vi "Update Plugin Status.vi"(8 "error in (no error)":errorcluster, 11 "CIF_UI in":refnum<class "CIF_UI.lvclass">) -> (0 "error out":errorcluster, 3 "CIF_UI out":refnum<class "CIF_UI.lvclass">)   [LabVIEW 2021, in "CIF_UI.lvclass"]
uses:
  CIF_UI.lvclass
  CIF_UI.lvclass/CIF_UI.ctl
  <vilib>/Utility/miscctls.llb/LVMapReplaceAction.ctl
  <vilib>/Utility/error.llb/Clear Errors.vi
  <vilib>/gRPC/LabVIEW gRPC Library/Client API/Close Client.vi
  CIFPluginManager/gRPC/CIF_Manager_Client_Wrapper/CIFManagerClientWrapper.lvlib
  CIFCore/Grpc/CIFCoreWrapper/CIFCoreWrapper.lvlib
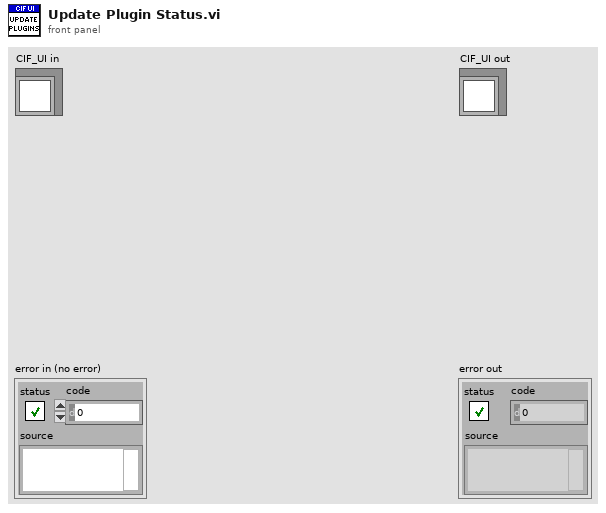
[diagram p1: front panel]
types:
  T1 = typedef "LVMapReplaceAction.ctl" = enum32{"Modify Entry only if found", "Add or Modify Entry", "Delete Entry"}
  T2 = typedef "CIF_UI.lvclass/Plugin Connection Map.ctl" = map{string, T3}
  T3 = typedef "CIF_UI.lvclass/Plugin Connections.ctl" = cluster{"gRPC ID":T4, "Plugin Info":T5}
  T4 = typedef "grpc-lvsupport-release.lvlib/grpcId.ctl" = u64
  T5 = typedef "CIFCoreCommon.lvlib/PluginInfo.ctl" = cluster{"Name":string, "Type":string, "grpc_port":i32, "Version":T6, "Node Status":T7}
  T6 = typedef "CIFCoreCommon.lvlib/Version Simple.ctl" = cluster{"Major":i32, "Minor":i32, "Fix":i32}
  T7 = typedef "CIFCoreCommon.lvlib/gRPC Reported Plugin Status.ctl" = cluster{"State":T8, "Timing Statistics (us)":T9, "FIFO Statistics (us)":T11, "error":T12, "Monitor Doubles":T13, "Monitor U64":T14, "Monitor I64":T15}
  T8 = typedef "CIFCoreCommon.lvlib/Plugin State.ctl" = enum32{"Null", "Creating", "Listening", "Running", "CleaningUp", "Destroying"}
  T9 = typedef "CIFCoreCommon.lvlib/Timing Statistics.ctl" = cluster{"Period":T10, "Wake Error":T10, "Execute":T10, "Housekeep":T10, "Idle":T10, "Cleanup":T10, "Custom 1 (custom units)":T10, "Custom 2 (custom units)":T10}
  T10 = typedef "CIFCoreCommon.lvlib/Timing Stats Base.ctl" = cluster{"Max":i64, "Avg":dbl, "Min":i64}
  T11 = typedef "CIFCoreCommon.lvlib/FIFO Statistics.ctl" = cluster{"From T0":T10, "From Previous Plugin":T10, "Output Error":T10}
  T12 = typedef "CIFCoreCommon.lvlib/Simple Error.ctl" = cluster{"status":bool, "code":i32}
  T13 = typedef "CIFCoreCommon.lvlib/Monitor Doubles.ctl" = cluster{"1":dbl, "2":dbl, "3":dbl, "4":dbl}
  T14 = typedef "CIFCoreCommon.lvlib/Monitor U64.ctl" = cluster{"1":u64, "2":u64, "3":u64, "4":u64}
  T15 = typedef "CIFCoreCommon.lvlib/Monitor I64.ctl" = cluster{"1":i64, "2":i64, "3":i64, "4":i64}
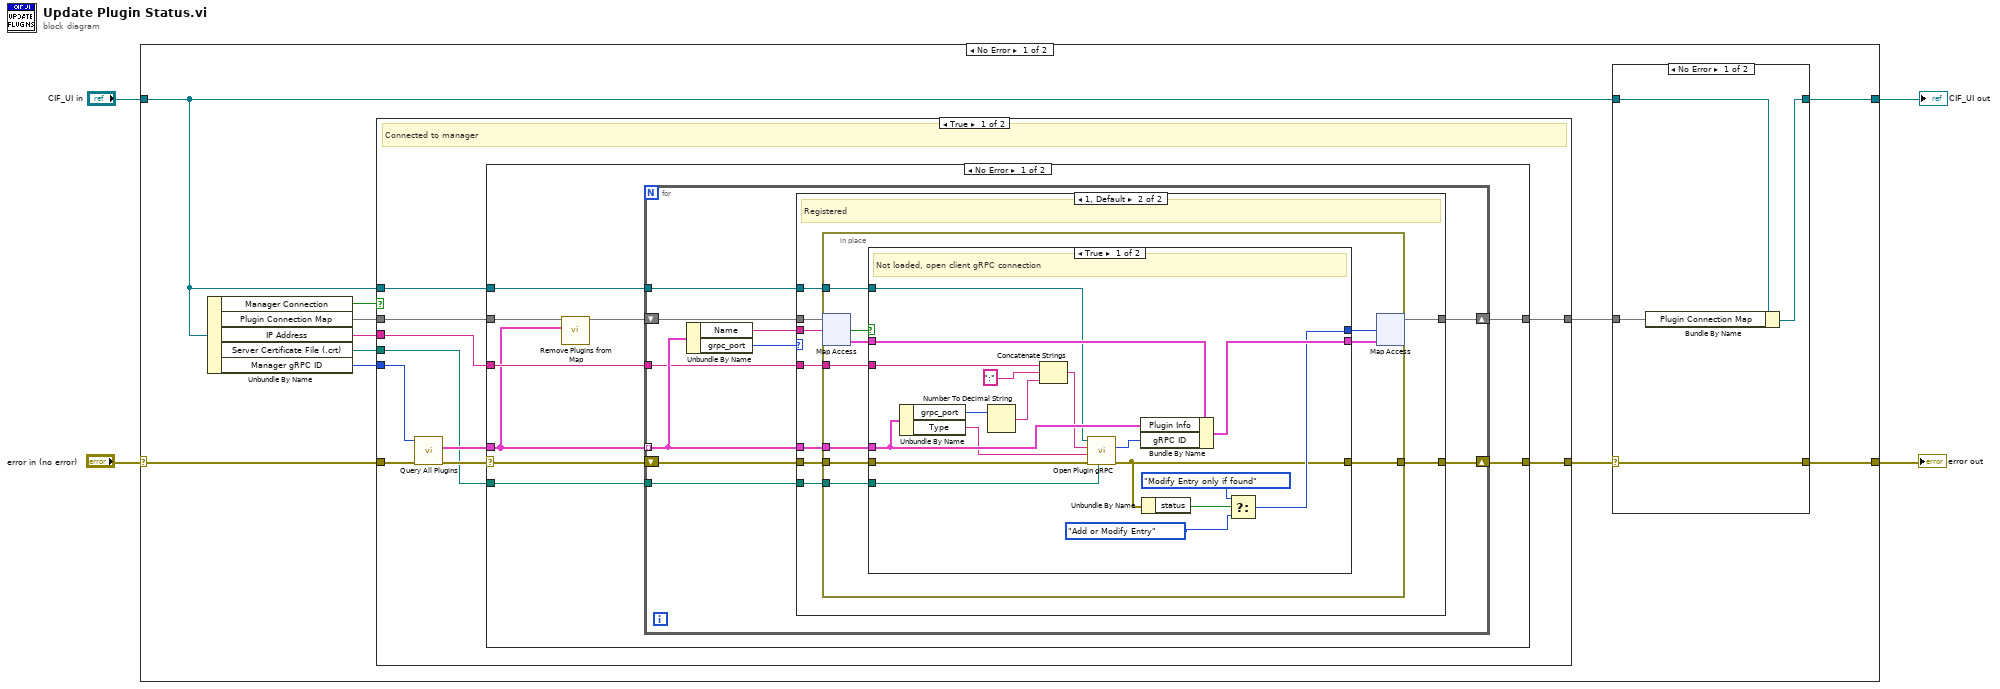
[diagram p0: block diagram]
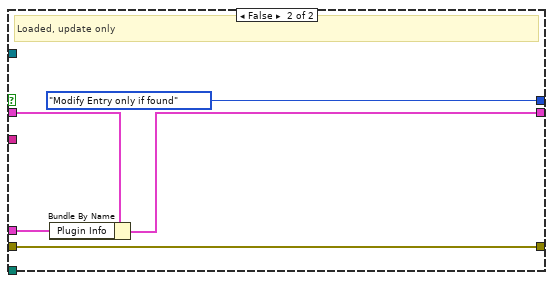
[diagram p4: hidden frame]
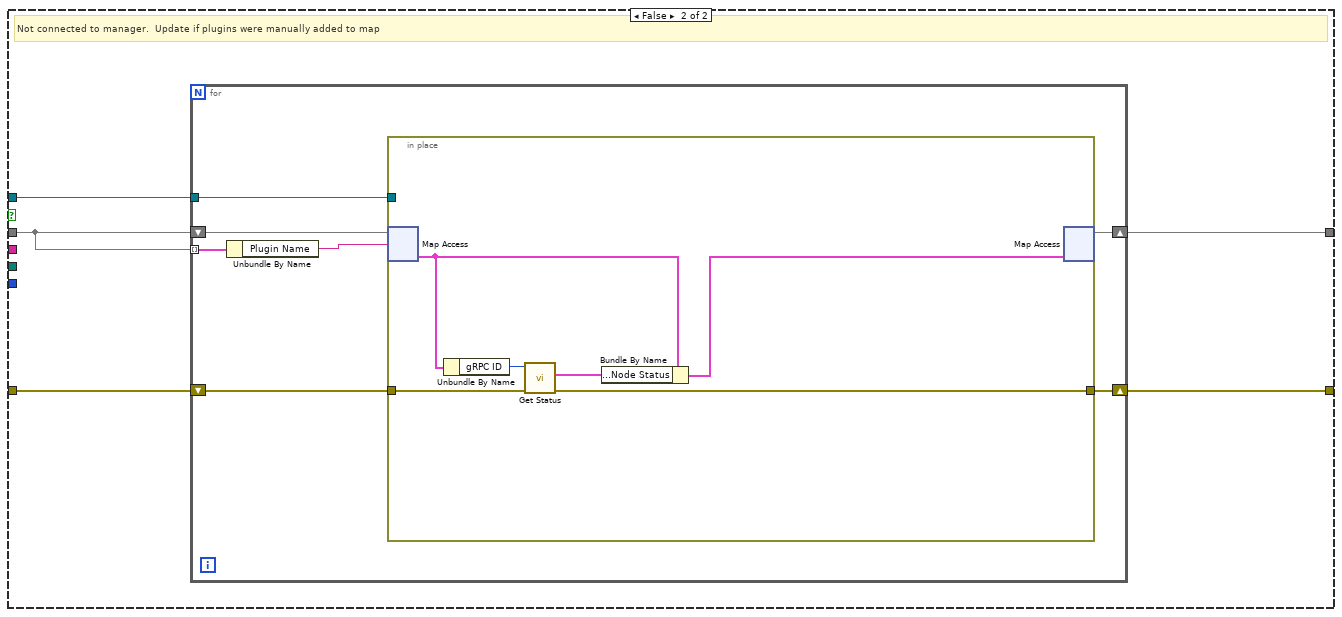
[diagram p6: hidden frame]
diagram:
  n1 = case shown="No Error" "error in (no error)" {
    selector: "error in (no error)" -> [w11 w116]
    tunnel: [w6 w116] -> w3
    tunnel: [w7 w115] -> w1
    tunnel: "CIF_UI in" -> [w9 w115]
    frame No Error {
      n2 = Unbundle By Name(w9) -> ("Manager Connection"=w10:bool, "Plugin Connection Map"=w15:T2, "IP Address"=w14:string, "Server Certificate File (.crt)"=w13:path, "Manager gRPC ID"=w12:T4)
      n3 = case shown="True" w10 {
        tunnel: w15 -> [w29 w97]
        tunnel: w14 -> [w28 _]
        tunnel: w13 -> [w27 _]
        tunnel: w12 -> [w26 _]
        tunnel: w11 -> [w25 w98]
        tunnel: [w22 w99] -> w5
        tunnel: w9 -> [w24 w101]
        tunnel: [w23 w100] -> w8
        frame True {
          # "Connected to manager"
          n4 = call "Query All Plugins.vi"("error in"=w25, "gRPC ID in"=w26) -> ("error out"=w31:errorcluster, "plugin_info"=w30:T5[])  [unwired: 7 in, 1 out]
          n5 = case shown="No Error" w31 {
            selector: w31 -> [w38 w96]
            tunnel: w30 -> [w32 _]
            tunnel: w29 -> [w34 w95]
            tunnel: w28 -> [w40 _]
            tunnel: w27 -> [w39 _]
            tunnel: [w37 w96] -> w22
            tunnel: [w36 w95] -> w23
            tunnel: w24 -> [w35 _]
            frame No Error {
              n6 = call "Remove Plugins from Map.vi"("plugin_info"=w32, "Plugin Connection Map in"=w34) -> ("Plugin Connection Map out"=w33:T2)  [unwired: 9 in]
              n7 = for {
                tunnel: w32 -> [w48] mode=indexing
                tunnel: w40 -> [w47]
                tunnel: w39 -> [w46]
                shift-right: [w43] -> w37
                shift-left: w38 -> [w45]
                shift-right: [w42] -> w36
                shift-left: w33 -> [w50]
                tunnel: w35 -> [w41]
                n8 = Unbundle By Name(w48) -> ("Name"=w49:string, "grpc_port"=w44:i32)
                n9 = case shown="1, Default" w44 {
                  tunnel: w50 -> [w52 w61]
                  tunnel: w49 -> [_ w60]
                  tunnel: w48 -> [_ w59]
                  tunnel: w47 -> [_ w58]
                  tunnel: w46 -> [_ w57]
                  tunnel: w45 -> [w51 w56]
                  tunnel: [w51 w55] -> w43
                  tunnel: [w52 w54] -> w42
                  tunnel: w41 -> [_ w53]
                  frame -1, 0 {
                    # "Not a valid port.  Not yet registered"
                  }
                  frame 1, Default {
                    # "Registered"
                    n10 = in-place {
                      in-place-border: w59 -> [w70]
                      in-place-border: w58 -> [w68]
                      in-place-border: w57 -> [w67]
                      in-place-border: w56 -> [w66]
                      in-place-border: [w63] -> w55
                      in-place-border: w53 -> [w62]
                      n11 = in-place-map #1(w61, w60) -> (w69:T3, w71:bool)  [unwired: 1 in]
                      n12 = case shown="True" w71 {
                        tunnel: w70 -> [w86 w93]
                        tunnel: w69 -> [w87 w94]
                        tunnel: w68 -> [w80 _]
                        tunnel: w67 -> [w78 _]
                        tunnel: w66 -> [w77 w90]
                        tunnel: [w85 w92] -> w65
                        tunnel: [w81 LVMapReplaceAction."Modify Entry only if found" ("action")] -> w64
                        tunnel: [w76 w90] -> w63
                        tunnel: w62 -> [w74 _]
                        frame True {
                          # "Not loaded, open client gRPC connection"
                          n13 = Unbundle By Name(w86) -> ("grpc_port"=w89:i32, "Type"=w72:string)
                          n14 = Number To Decimal String(number=w89) -> (decimal integer string=w88:string)  [unwired: 1 in]
                          n15 = Concatenate Strings(w80, ":" ("regular expression"), w88) -> (w73:string)
                          n16 = call-dynamic "Open Plugin gRPC.vi"("Server Certificate File (.crt)"=w78, "error in (no error)"=w77, "Type"=w72, "address"=w73, "CIF_UI in"=w74) -> ("error out"=w76:errorcluster, "gRPC ID Out"=w75:T4)  [unwired: 4 in, 1 out]
                          n17 = Bundle By Name(cluster=w87, "Plugin Info"=w86, "gRPC ID"=w75) -> (w85:T3)
                          n18 = Unbundle By Name(w76) -> ("status"=w84:bool)
                          n19 = Select(t=LVMapReplaceAction."Modify Entry only if found", s=w84, f=LVMapReplaceAction."Add or Modify Entry" ("action")) -> (s? t:f=w81:T1)
                        }
                        frame False {
                          # "Loaded, update only"
                          n20 = Bundle By Name(cluster=w94, "Plugin Info"=w93) -> (w92:T3)
                        }
                      }
                      n21 = in-place-map #1(w65, w64) -> (w54:T2)  [unwired: 2 out]
                    }
                  }
                }
              }
            }
            frame Error {
            }
          }
        }
        frame False {
          # "Not connected to manager.  Update if plugins were manually added to map"
          n22 = for {
            shift-right: [w106] -> w99
            shift-left: w98 -> [w107]
            shift-right: [w105] -> w100
            shift-left: w97 -> [w108]
            tunnel: w101 -> [w104]
            tunnel: w97 -> [w103] mode=indexing
            n23 = Unbundle By Name(w103) -> ("Plugin Name"=w102:string)
            n24 = in-place {
              in-place-border: w107 -> [w113]
              in-place-border: [w112] -> w106
              in-place-border: w104 -> [_]
              n25 = in-place-map #2(w108, w102) -> (w114:T3)  [unwired: 1 in, 1 out]
              n26 = Unbundle By Name(w114) -> ("gRPC ID"=w110:T4)
              n27 = call "Get Status.vi"("error in"=w113, "gRPC ID"=w110) -> ("error out"=w112:errorcluster, "Node Status"=w109:T7)  [unwired: 7 in, 1 out]
              n28 = Bundle By Name(cluster=w114, "Plugin Info.Node Status"=w109) -> (w111:T3)
              n29 = in-place-map #2(w111) -> (w105:T2)  [unwired: 1 in, 2 out]
            }
          }
        }
      }
      n30 = case shown="No Error" w5 {
        selector: w5 -> [w16 w20]
        tunnel: w8 -> [w19 _]
        tunnel: w9 -> [w18 w21]
        tunnel: [w17 w21] -> w7
        tunnel: [w16 w20] -> w6
        frame No Error {
          n31 = Bundle By Name(cluster=w18, "Plugin Connection Map"=w19) -> (w17:refnum<class "CIF_UI.lvclass">)
        }
        frame Error {
        }
      }
    }
    frame Error {
    }
  }
  "error out" <- w3
  "CIF_UI out" <- w1
